vi "Init.vi"(8 "error in (no error)":errorcluster, 10 "Pause":bool, 11 "Cmd Q":refnum<queue>) -> (0 "error out":errorcluster)   [LabVIEW 2020, in "FormulaG.lvlib" / "Pause Cmd.lvclass"]
uses:
  Pause Cmd.lvclass
  Command/Command.lvclass
  C:/dev/SummerOfLabVIEW/sol-formulag/ProjectTemplates/Source/SummerOfLabVIEW/FormulaG/template/FormulaG/Command/Command.lvclass
  Pause Cmd.lvclass/Pause Cmd.ctl
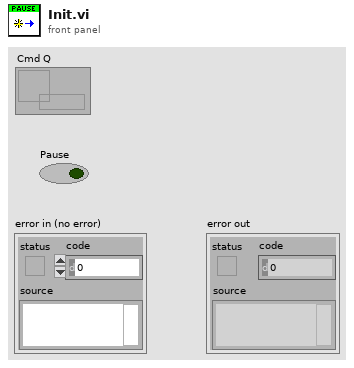
[diagram p1: front panel]
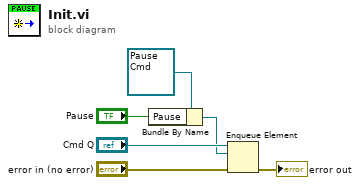
[diagram p0: block diagram]
diagram:
  n1 = Bundle By Name(cluster=refnum<class "Pause Cmd.lvclass"> refnum ("Pause Cmd in"), "Pause"="Pause") -> (w1:refnum<class "Pause Cmd.lvclass">)
  n2 = Enqueue Element(queue="Cmd Q", element=w1, error in (no error)="error in (no error)") -> (error out=→"error out":errorcluster)  [unwired: 1 in, 2 out]
